vi "pxi test.vi"() -> ()   [LabVIEW 2023]
uses:
  PXI-5441_class/PXI-5441.lvclass
panel:
  in  "Error":bool
  in  "Disconnect Button":bool
  in  "Connect Button":bool
  in  "Resource Name":refnum<k15>
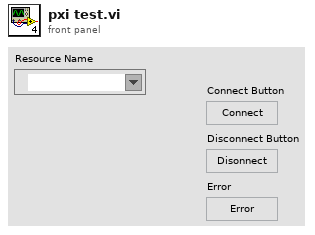
[diagram p1: front panel]
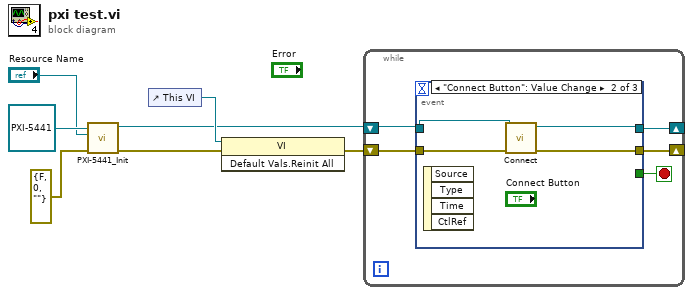
[diagram p0: block diagram]
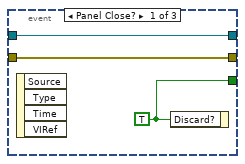
[diagram p2: hidden frame]
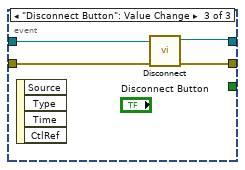
[diagram p3: hidden frame]
diagram:
  n1 = call "PXI-5441_Init.vi"("Error In"=errorcluster {"status"=FALSE, "code"=0, "source"=""}, "Resource Name"="Resource Name", "Object in"=refnum<class "PXI-5441.lvclass"> refnum ("PXI-5441.lvlib:PXI-5441")) -> ("Error Out"=w2:errorcluster, "object out"=w3:refnum<class "PXI-5441.lvclass">)  [unwired: 7 in]
  n2 = control-ref of="This VI"() -> (w4:refnum<vi>)
  n3 = invoke class="VI" method="Default Vals.Reinit All"(reference=w4, error in=w2) -> (error out=w1:errorcluster)  [unwired: 1 in, 2 out]
  n4 = while {
    shift-right: [w9] -> _
    shift-left: w1 -> [w11]
    shift-right: [w8] -> _
    shift-left: w3 -> [w12]
    stop <- w10 stop-if-true
    n5 = event shown="[1] \"Connect Button\": Value Change" {
      selector: _ -> [_ _ _]
      dyn-events: _ -> [_ _ _]
      timeout: _ -> [_ _ _]
      tunnel: w12 -> [w14 w19 w22]
      tunnel: [w14 w18 w21] -> w8
      tunnel: [w15 _ _] -> w10
      tunnel: w11 -> [w13 w17 w23]
      tunnel: [w13 w16 w20] -> w9
      event Panel Close? {
        w15 = TRUE ("Discard?")
        n6 = event-data() -> ()  [unwired: 1 in, 4 out]
        n7 = event-data("Discard?"=w15) -> ()  [unwired: 1 in, 1 out]
      }
      event "Connect Button": Value Change {
        n8 = event-data() -> ()  [unwired: 1 in, 4 out]
        n9 = call-dynamic "Connect.vi"("Error In"=w17, "object in"=w19) -> ("Error Out"=w16:errorcluster, "object out"=w18:refnum<class "PXI-5441.lvclass">)  [unwired: 8 in]
      }
      event "Disconnect Button": Value Change {
        n10 = event-data() -> ()  [unwired: 1 in, 4 out]
        n11 = call "Disconnect.vi"("error in (no error)"=w23, "PXI-5441 in"=w22) -> ("error out"=w20:errorcluster, "PXI-5441 out"=w21:refnum<class "PXI-5441.lvclass">)  [unwired: 8 in]
      }
    }
  }
